vi "ReadVoltage.vi"(8 "Error In":errorcluster, 11 "reference in":refnum<class "VdAnalogInput.lvclass">) -> (0 "Error Out":errorcluster, 2 "Voltage":dbl, 3 "reference out":refnum<class "VdAnalogInput.lvclass">)   [LabVIEW 2020, in "VdAnalogInput.lvclass"]
uses:
  VdAnalogInput.lvclass
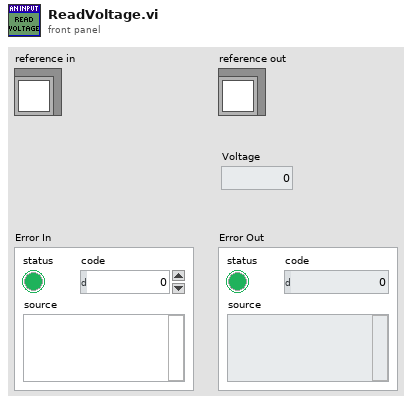
[diagram p1: front panel]
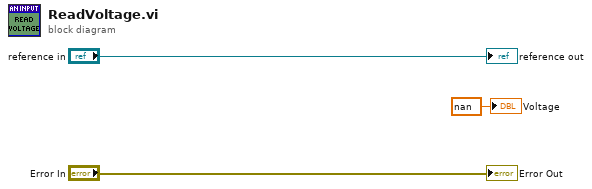
[diagram p0: block diagram]
diagram:
  "Error Out" <- "Error In"
  "reference out" <- "reference in"
  "Voltage" <- nan ("Voltage")
